vi "Process.vi"(8 "error in":errorcluster, 11 "Inst.Krohn-Hite-7008":refnum<class "Inst.Krohn-Hite-7008.lvclass">) -> (0 "error out":errorcluster, 3 "Inst.Krohn-Hite-7008 out":refnum<class "Inst.Krohn-Hite-7008.lvclass">)   [LabVIEW 2019, in "Inst.Krohn-Hite-7008.lvclass"]
doc: "---------------------------------------------------------------\nJKI State Machine Objects™\nhttp://jki.net/state-machine-objects/\nCopyright (C) 2005-2015, JKI <info@jki.net>\nALL RIGHTS RESERVED"
uses:
  Inst.Krohn-Hite-7008.lvclass
  C:/Program Files (x86)/National Instruments/LabVIEW 2019/vi.lib/JKI/JKI SMO/SMO/SMO.lvclass
  C:/Program Files (x86)/National Instruments/LabVIEW 2019/user.lib/LevyLab/Instrument Framework/Instrument/Instrument.lvclass
  Typedefs/Inst.Krohn-Hite-7008.Commands--Enum.ctl
  Typedefs/PrivateEvents--Inst.Krohn-Hite-7008.MessageToProcess.ctl
  <userlib>/LevyLab/RemoteControl/Typedefs/Message--Cluster.ctl
  <vilib>/JKI/JKI SMO/SMO/SMO.lvclass/SMO.ctl
  Inst.Krohn-Hite-7008.lvclass/Inst.Krohn-Hite-7008.ctl
  Typedefs/Inst.Krohn-Hite-7008.ProtectedCommands--Enum.ctl
  ef847fcc-ae38-4c9a-a9d7-f0d56e5c7fa0.vi
  c2686cc3-20e9-4710-a87a-2e2b9cb24138.vi
  <vilib>/JKI/JKI SMO/SMO/Private/ReftoDVR--SMO.vi
  <vilib>/Utility/Data Type/Get Type Information.vi
  <vilib>/Utility/Data Type/Get Numeric Information.vi
  <userlib>/_OpenG.lib/lvdata/lvdata.llb/Unwrap VVariant__ogtk.vi
  <userlib>/LevyLab/Instrument Framework/Instrument Types/Amplifier/Instrument.Amplifier.lvclass
  <vilib>/JKI/JKI SMO/SMO/SMO.lvclass
  <userlib>/LevyLab/Instrument Framework/Instrument/Instrument.lvclass
  <userlib>/LevyLab/RemoteControl/RemoteControl.lvclass
  KH7008/KH7008.lvlib
  <userlib>/LevyLab/Configuration/Debug.lvlib
panel:
  out "Status":string
  out "State History":string
  # "Instrument.Krohn-Hite-7008"
  # "Instrument.Krohn-Hite-7008"
  # "For instructions on how to use the JKI State Machine Objects, examples and video tutorials, visit:\nhttp://jki.net/state-machine-objects/\n\nJKI State Machine Objects™\nhttp://jki.net/state-machine-objects/\nCopyright (C) 2005-2015, JKI <info@jki.net>\nALL RIGHTS RESERVED"
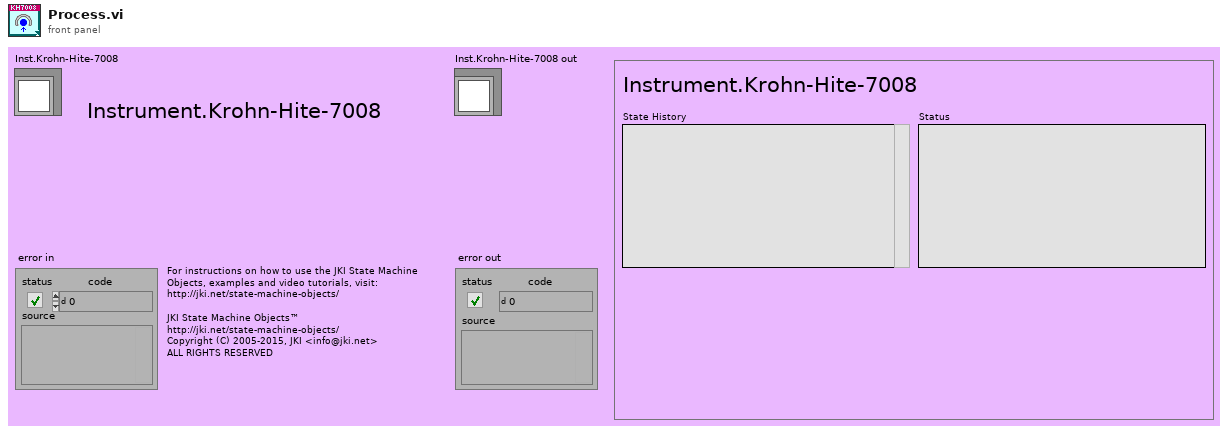
[diagram p1: front panel]
types:
  T1 = typedef "Inst.Krohn-Hite-7008.lvclass/Inst.Krohn-Hite-7008.Commands--Enum.ctl" = enum16{"getChannel", "getAllChannels", "setChannel", "setAllChannels"}
  T2 = enum32{"invalid app kind", "Development System", "Run Time System", "Student Edition", "Embedded LabVIEW", "Evaluation", "Custom"}
  T3 = enum32{"Invalid", "Standard", "Closed", "Hidden", "Minimized", "Maximized"}
  T4 = typedef "Inst.Krohn-Hite-7008.lvclass/Inst.Krohn-Hite-7008.ProtectedCommands--Enum.ctl" = enum16{"Update allChannelProperties", "Update device", "Set SR"}
  T5 = typedef "Inst.Krohn-Hite-7008.lvclass/PrivateEvents--Inst.Krohn-Hite-7008.MessageToProcess.ctl" = cluster{"Message":T6}
  T6 = typedef "RemoteControl.lvclass/Message--Cluster.ctl" = cluster{"Command":string, "Data":variant, "ID":string}
  T7 = cluster{"Core":cluster{"Current VI Reference":refnum<vi>, "Close Panel on Exit?":bool, "Last Error":cluster{"error":errorcluster, "previous state":string, "remaining states":string}, "Shutdown?":bool}, "SelfRef":refnum<class "Inst.Krohn-Hite-7008.lvclass">, "Running Step":i32, "sequence":string[], "MessageToProcess":T5, "UI Behavior":string, "wait":u32}
  T8 = cluster{"Current VI Reference":refnum<vi>, "Close Panel on Exit?":bool, "Last Error":cluster{"error":errorcluster, "previous state":string, "remaining states":string}, "Shutdown?":bool}
  T9 = typedef "Debug.lvlib/Attribute.Debug.lvclass/DebugBehavior.ctl" = enum16{"Normal", "Debug"}
  T10 = typedef "SMO.lvclass/Protected Events.ctl" = cluster{"StopProcesses":refnum<user-event>, "AbortProcesses":refnum<user-event>, "Config Changed":refnum<user-event>, "Dependency":refnum<user-event>}
  T11 = typedef "KH7008.lvlib/allChannelProperties--Array.ctl" = T12[]
  T12 = typedef "KH7008.lvlib/channelProperties--Cluster.ctl" = cluster{"channel":T13, "gain":T14, "input":T15, "shunt":T16, "couple":T17, "filter":T18}
  T13 = typedef "KH7008.lvlib/channel--numeric.ctl" = u16
  T14 = typedef "KH7008.lvlib/gain--enum.ctl" = enum16{"1", "10", "100", "1000"}
  T15 = typedef "KH7008.lvlib/input--enum.ctl" = enum16{"OFF", "SE+", "SE-", "DIFF"}
  T16 = typedef "KH7008.lvlib/shunt--enum.ctl" = enum16{"Open", "50", "500", "5k", "50k", "10M"}
  T17 = typedef "KH7008.lvlib/couple--enum.ctl" = enum16{"AC", "DC"}
  T18 = typedef "KH7008.lvlib/filter--enum.ctl" = enum16{"OFF", "ON"}
  T19 = typedef "Inst.Krohn-Hite-7008.lvclass/Inst.Krohn-Hite-7008.getAll--Cluster.ctl" = cluster{"device_id":string, "model":string, "allChannelProperties_json":string, "allChannelProperties":T11}
  T20 = typedef "Inst.Krohn-Hite-7008.lvclass/getAllChannelsDatabase--Cluster.ctl" = cluster{"device_id":string, "channel":u32, "gain":string, "input":string, "shunt":string, "couple":string, "filter":string}
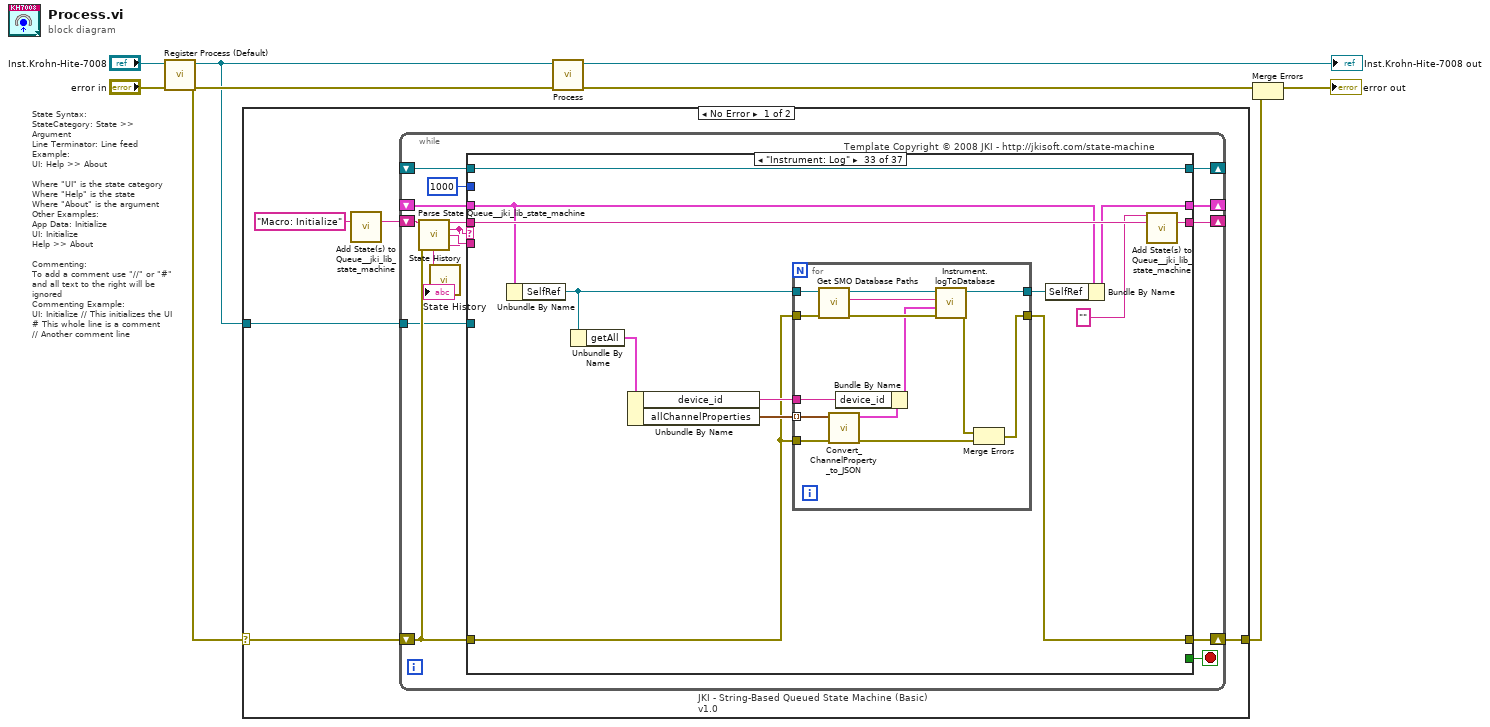
[diagram p0: block diagram]
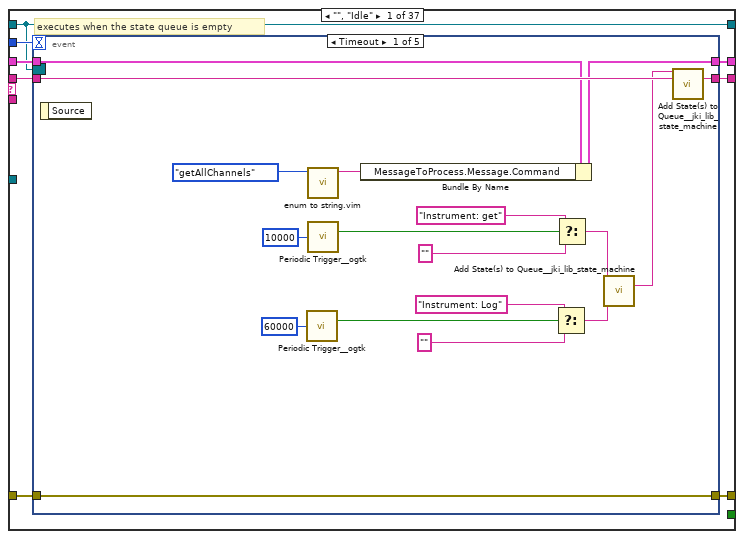
[diagram p2: hidden frame]
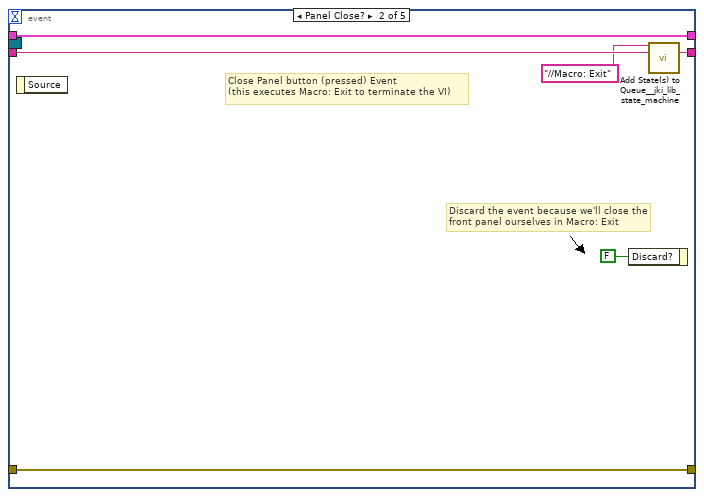
[diagram p3: hidden frame]
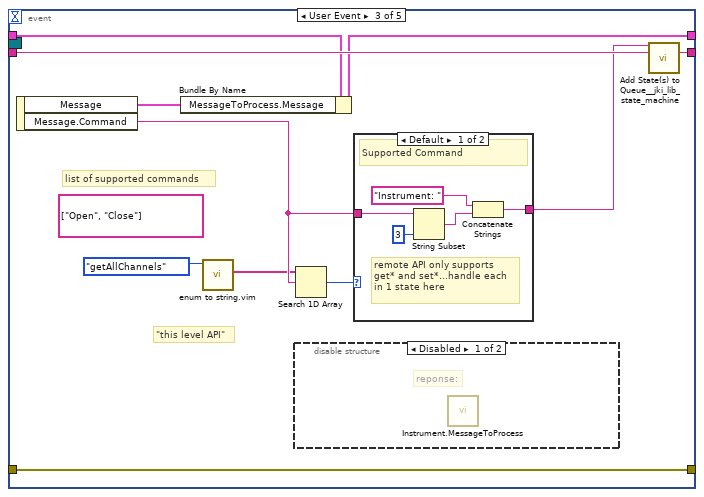
[diagram p4: hidden frame]
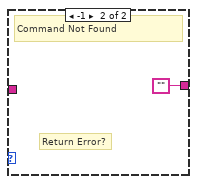
[diagram p6: hidden frame]
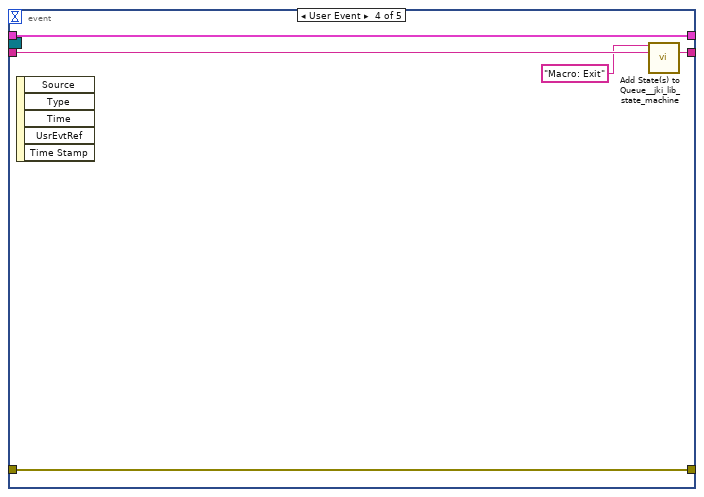
[diagram p7: hidden frame]
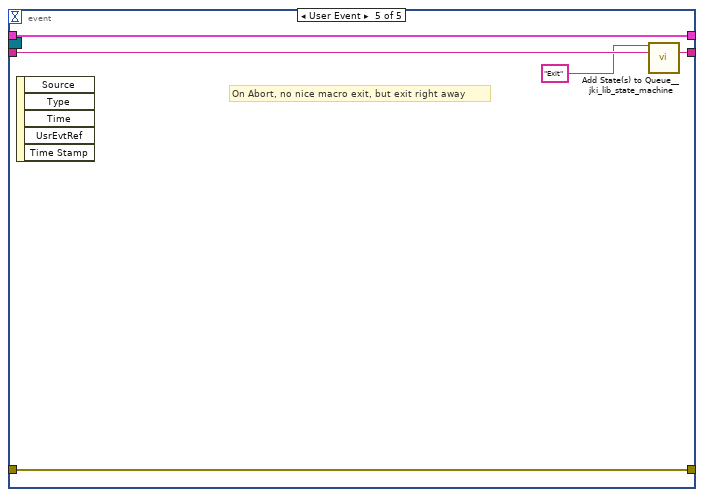
[diagram p8: hidden frame]
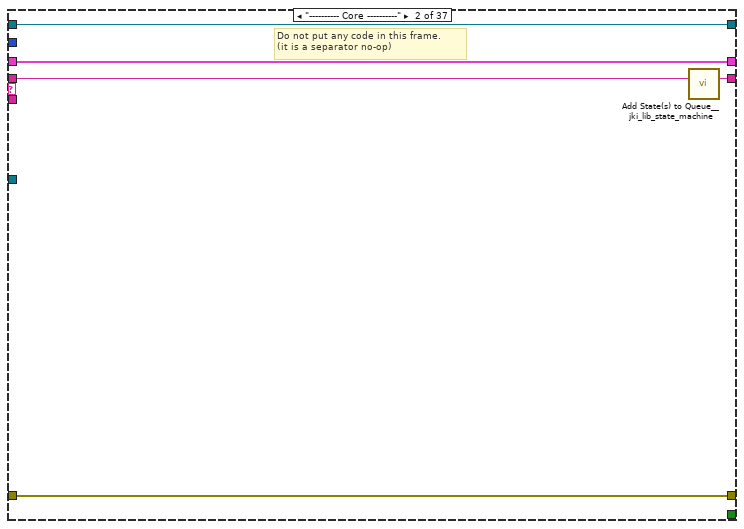
[diagram p9: hidden frame]
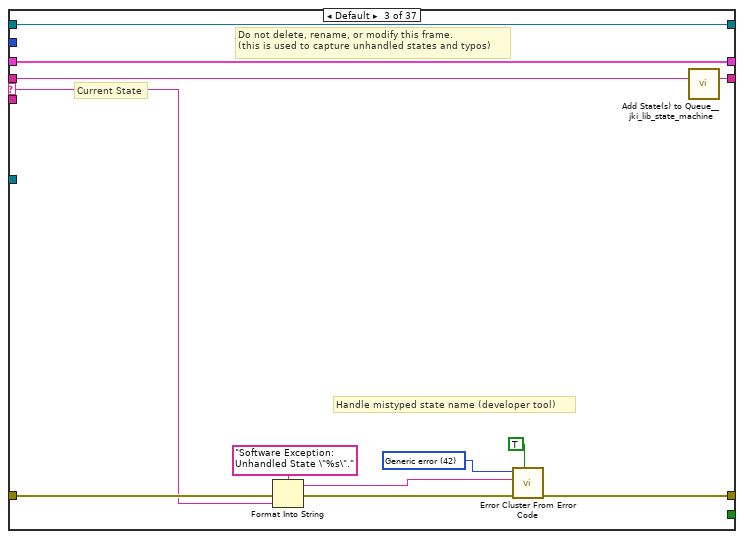
[diagram p10: hidden frame]
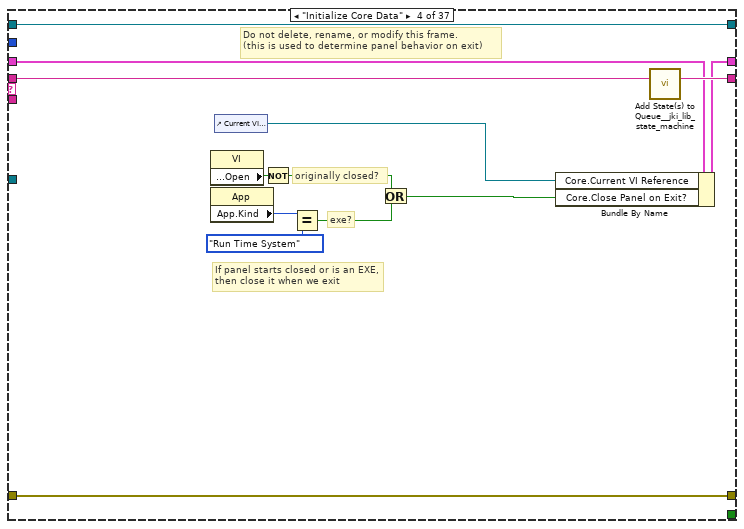
[diagram p11: hidden frame]
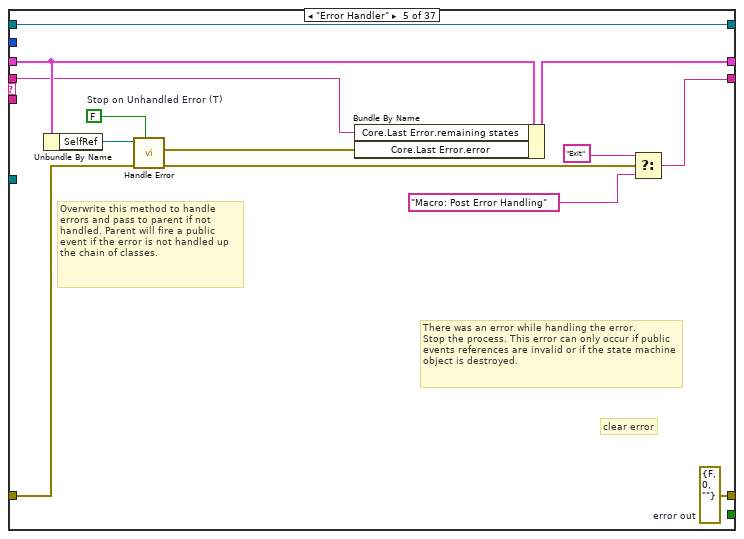
[diagram p12: hidden frame]
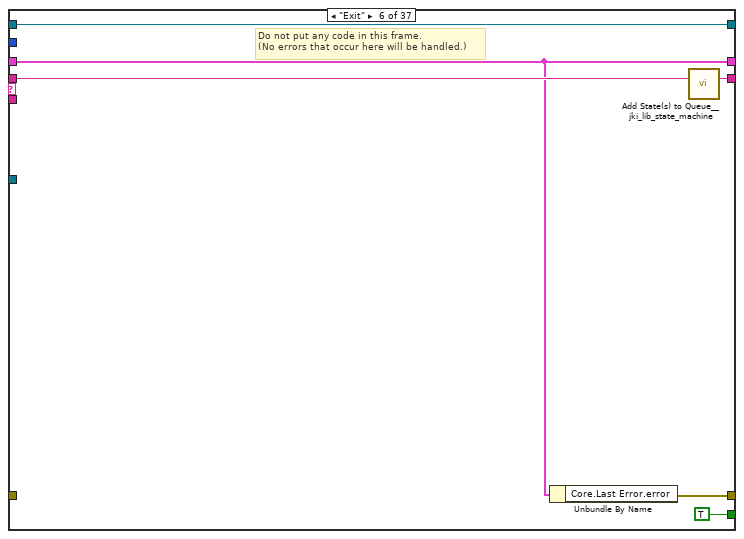
[diagram p13: hidden frame]
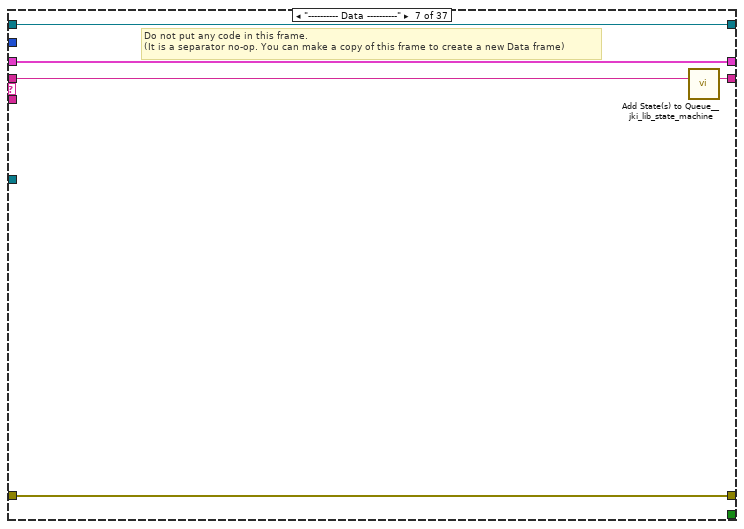
[diagram p14: hidden frame]
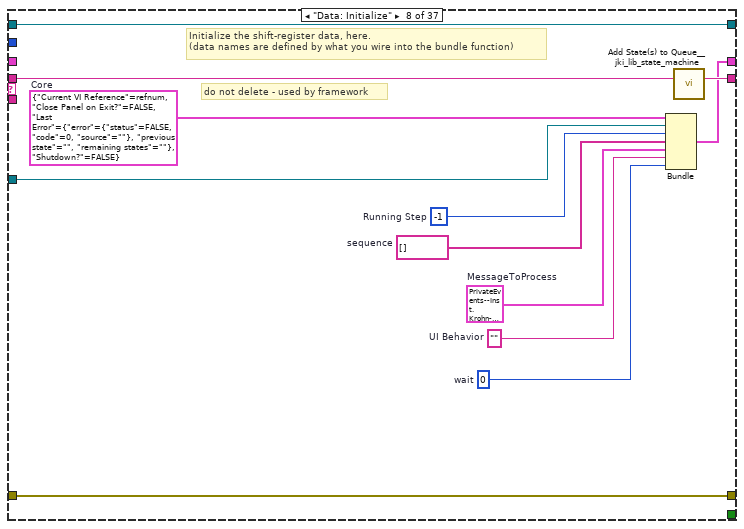
[diagram p15: hidden frame]
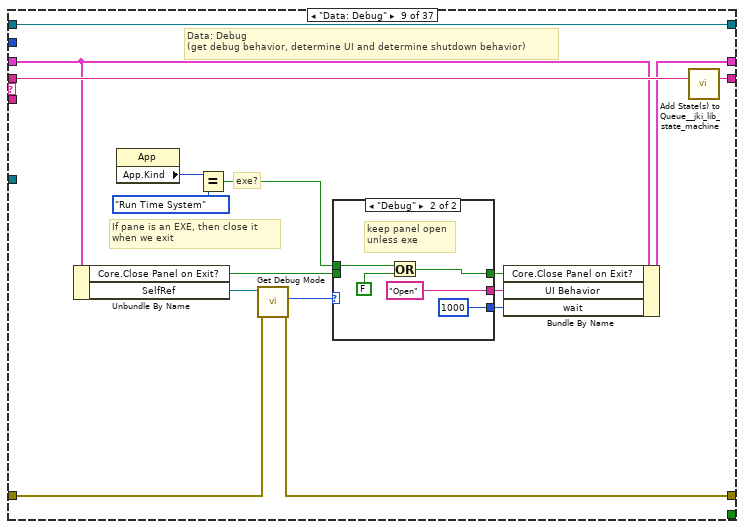
[diagram p16: hidden frame]
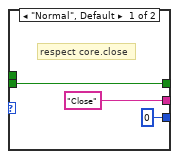
[diagram p17: hidden frame]
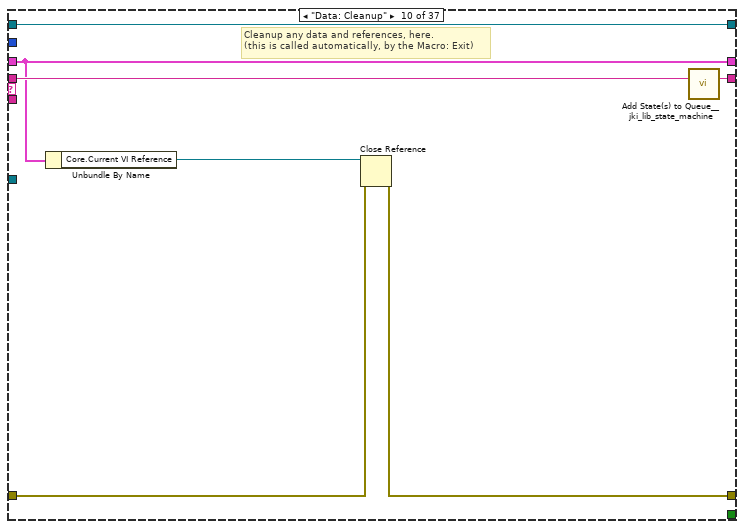
[diagram p18: hidden frame]
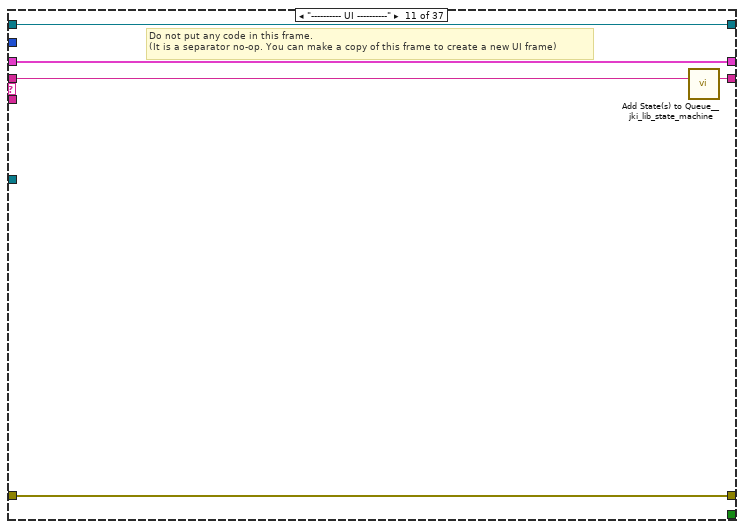
[diagram p19: hidden frame]
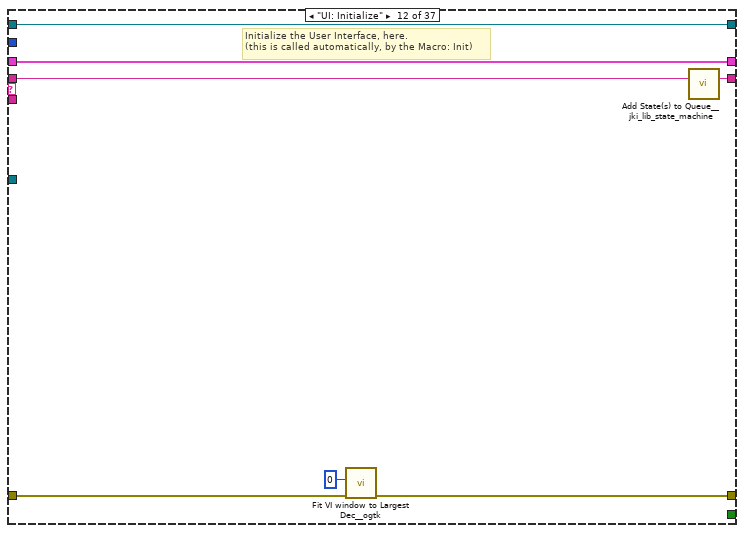
[diagram p20: hidden frame]
diagram:
  # "State Syntax:\nStateCategory: State >> Argument\nLine Terminator: Line feed\nExample:\nUI: Help >> About\n\nWhere \"UI\" is the state category\nWhere \"Help\" is the state\nWhere \"About\" is the argument\nOther Examples:\nApp Data: Initialize\nUI: Initialize\nHelp >> About\n\nCommenting:\nTo add a comment use \"//\" or \"#\" and all text to the right will be ignored\nCommenting Example:\nUI: Initialize // This initializes the UI\n# This whole line is a comment\n// Another comment line"
  n1 = call <vilib>:"Register Process (Default).vi"("error in (no error)"="error in", "SMO"="Inst.Krohn-Hite-7008") -> ("error out"=w5:errorcluster, "SelfRef"=w4:refnum<class "Inst.Krohn-Hite-7008.lvclass">)  [unwired: 8 in]
  n2 = case shown="No Error" w5 {
    selector: w5 -> [w10 w522]
    tunnel: w4 -> [w11 _]
    tunnel: [w9 w522] -> w1
    frame No Error {
      n3 = call <vilib>:"Add State(s) to Queue__jki_lib_state_machine.vi"("State(s) in (\"\")"="Macro: Initialize") -> ("States Out"=w13:string)  [unwired: 14 in]
      n4 = while "JKI - String-Based Queued State Machine (Basic) v1.0" {
        shift-right: [w22] -> _
        shift-left: _ -> [w21]
        shift-right: [w25] -> w9
        shift-left: w10 -> [w19]
        shift-right: [w24] -> _
        shift-left: w13 -> [w26]
        tunnel: w11 -> [w18]
        shift-right: [w17] -> _
        shift-left: _ -> [w16]
        stop <- w23 stop-if-true
        # "Template Copyright © 2008 JKI - http://jkisoft.com/state-machine"
        n5 = call <vilib>:"Parse State Queue__jki_lib_state_machine.vi"("State Queue"=w26, "Error In (no error)"=w19) -> ("Remaining States"=w28:string, "Current State"=w15:string, "Arguments"=w27:string)  [unwired: 11 in]
        n6 = call <userlib>:"State History.vi"("Current State"=w15) -> ("History"=→"State History":string)  [unwired: 10 in]
        n7 = case shown="\"Instrument: Log\"" w15 {
          selector: w15 -> [_ _ w94 _ _ _ _ _ _ _ _ _ _ _ _ _ _ _ _ _ _ _ _ _ _ _ _ _ _ _ _ _ _ _ _ _ _]
          tunnel: w28 -> [w36 w92 w98 w117 w122 w136 w141 w153 w169 w184 w189 w196 w203 w219 w251 w260 w268 w274 _ w317 w332 w337 w348 w355 w360 w373 w379 w386 w395 w409 w428 w455 w468 w491 w496 w502 w521]
          tunnel: w27 -> [_ _ _ _ _ _ _ _ _ _ _ _ w197 w213 _ _ _ _ _ _ _ _ _ _ _ _ _ _ _ _ _ _ _ _ _ w497 w505]
          tunnel: w21 -> [w34 w89 w96 w108 w126 w132 w138 _ w157 w179 w186 w194 w201 w215 w248 w257 w264 w271 w277 w307 w322 w334 w345 w352 w357 w366 w377 w381 w391 w405 w424 w451 w464 w487 w492 w498 w511]
          tunnel: [w33 w90 w100 w114 w127 w131 w139 w145 w156 w180 w187 w191 w198 w216 w249 w252 w266 w272 w285 w315 w318 w335 w339 w350 w358 w369 w375 w383 w388 w400 w420 w447 w459 w484 w493 w499 w513] -> w25
          tunnel: w19 -> [w32 w90 w99 w114 w128 _ w139 w145 w155 w181 w187 w190 w199 w217 w249 w252 w266 w272 w285 w315 w318 w335 w340 w349 w358 w363 w375 w383 w389 w399 w419 w448 w456 w483 w493 w499 w507]
          tunnel: [w35 w91 w97 w116 w118 w135 w140 w152 w168 w183 w188 w195 w202 w218 w250 w259 w267 w273 w286 w316 w331 w336 w347 w354 w359 w372 w378 w385 w394 w408 w427 w454 w467 w490 w495 w501 w520] -> w24
          tunnel: [_ _ _ _ _ TRUE _ _ _ _ _ _ _ _ _ _ _ _ _ _ _ _ _ _ _ _ _ _ _ _ _ _ _ _ _ _ _] -> w23
          tunnel: [w31 w89 w96 w115 w125 w132 w138 w151 w158 w179 w186 w194 w201 w215 w248 w257 w264 w271 w278 w308 w322 w334 w345 w352 w357 w366 w377 w382 w392 w406 w425 w452 w465 w488 w492 w498 w510] -> w22
          tunnel: 1000 ("Timeout") -> [w30 _ _ _ _ _ _ _ _ _ _ _ _ _ _ _ _ _ _ _ _ _ _ _ _ _ _ _ _ _ _ _ _ _ _ _ _]
          tunnel: w18 -> [_ _ _ _ _ _ _ w146 _ _ _ _ _ _ _ _ _ _ _ _ _ _ _ _ _ _ _ _ _ _ _ _ _ _ _ _ _]
          tunnel: [w29 w88 w93 w105 w130 w133 w137 w150 w167 w178 w185 w193 w200 w212 w247 w258 w265 w270 w284 w314 w327 w333 w346 w353 w356 w371 w376 w384 w393 w407 w426 w453 w466 w489 w494 w500 w519] -> w17
          tunnel: w16 -> [w29 w88 w93 w105 w130 w133 w137 w150 w167 w178 w185 w193 w200 w212 w247 w258 w265 w270 w284 w314 w327 w333 w346 w353 w356 _ w376 w384 w393 w407 w426 w453 w466 w489 w494 w500 w519]
          frame "", "Idle" {
            # "executes when the state queue is empty"
            n8 = event shown="[0] Timeout" {
              selector: w29 -> [_ _ _ _ _]
              dyn-events: _ -> [_ _ _ _ _]
              timeout: w30 -> [_ _ _ _ _]
              tunnel: w36 -> [w54 w60 w71 w82 w87]
              tunnel: [w53 w59 w70 w81 w86] -> w35
              tunnel: w34 -> [w48 w57 w64 w79 w84]
              tunnel: [w52 w58 w69 w80 w85] -> w33
              tunnel: w32 -> [w52 w58 w69 w80 w85]
              tunnel: [w49 w57 w65 w79 w84] -> w31
              event Timeout {
                n9 = event-data() -> ()  [unwired: 1 in, 1 out]
                n10 = call <userlib>:"Periodic Trigger__ogtk.vi"("time (ms)"=u32 60000) -> ("Triggered"=w40:bool)  [unwired: 12 in, 2 out]
                n11 = call "enum to string.vim"("enum in"=Inst.Krohn-Hite-7008.Commands--Enum."getAllChannels" ("Commands")) -> ("string out"=w51:string)  [unwired: 9 in, 1 out]
                n12 = call <userlib>:"Periodic Trigger__ogtk.vi"("time (ms)"=u32 10000) -> ("Triggered"=w47:bool)  [unwired: 12 in, 2 out]
                n13 = Bundle By Name(cluster=w48, "MessageToProcess.Message.Command"=w51) -> (w49:T7)
                n14 = Select(t="Instrument: Log", s=w40, f="") -> (s? t:f=w39:string)
                n15 = Select(t="Instrument: get", s=w47, f="") -> (s? t:f=w38:string)
                n16 = call <vilib>:"Add State(s) to Queue__jki_lib_state_machine.vi"("State(s) in Front (\"\")"=w38, "State(s) at Back (\"\")"=w39) -> ("States Out"=w37:string)  [unwired: 13 in]
                n17 = call <vilib>:"Add State(s) to Queue__jki_lib_state_machine.vi"("State(s) in Front (\"\")"=w37, "State(s) in (\"\")"=w54) -> ("States Out"=w53:string)  [unwired: 13 in]
              }
              event Panel Close? {
                # "Discard the event because we'll close the front panel ourselves in Macro: Exit"
                # "Close Panel button (pressed) Event\n(this executes Macro: Exit to terminate the VI)"
                n18 = event-data() -> ()  [unwired: 1 in, 1 out]
                n19 = event-data("Discard?"=FALSE) -> ()  [unwired: 1 in, 1 out]
                n20 = call <vilib>:"Add State(s) to Queue__jki_lib_state_machine.vi"("State(s) in Front (\"\")"="//Macro: Exit", "State(s) in (\"\")"=w60) -> ("States Out"=w59:string)  [unwired: 13 in]
              }
              event User Event {
                (unwired) string[] ["Open", "Close"]
                # "\"this level API\""
                # "list of supported commands"
                n21 = event-data() -> ("Message"=w63:T6, "Message.Command"=w66:string)  [unwired: 1 in]
                n22 = Bundle By Name(cluster=w64, "MessageToProcess.Message"=w63) -> (w65:T7)
                n23 = call "enum to string.vim"("enum in"=Inst.Krohn-Hite-7008.Commands--Enum."getAllChannels" ("Commands")) -> ("strings out"=w61:string[])  [unwired: 9 in, 1 out]
                n24 = disable-structure shown="Disabled" {
                  frame Disabled {
                    # "reponse:"
                    n25 = call <userlib>:"Instrument.MessageToProcess.vi"() -> ()  [unwired: 10 in, 2 out]
                  }
                  frame Enabled {
                  }
                }
                n26 = Search 1D Array(1D array=w61, element=w66) -> (index of element=w68:i32)  [unwired: 1 in]
                n27 = case shown="Default" w68 {
                  tunnel: [w76 "" ("Empty String Constant")] -> w67
                  tunnel: w66 -> [w72 _]
                  frame Default {
                    # "remote API only supports\nget* and set*...handle each \nin 1 state here"
                    # "Supported Command"
                    n28 = String Subset(string=w72, length (rest)=3 ("length (rest)")) -> (substring=w73:string)  [unwired: 1 in]
                    n29 = Concatenate Strings("Instrument: ", w73) -> (w76:string)
                  }
                  frame -1 {
                    # "Return Error?"
                    # "Command Not Found"
                  }
                }
                n30 = call <vilib>:"Add State(s) to Queue__jki_lib_state_machine.vi"("State(s) in Front (\"\")"=w67, "State(s) in (\"\")"=w71) -> ("States Out"=w70:string)  [unwired: 13 in]
              }
              event User Event {
                n31 = event-data() -> ()  [unwired: 1 in, 5 out]
                n32 = call <vilib>:"Add State(s) to Queue__jki_lib_state_machine.vi"("State(s) in Front (\"\")"="Macro: Exit", "State(s) in (\"\")"=w82) -> ("States Out"=w81:string)  [unwired: 13 in]
              }
              event User Event {
                # "On Abort, no nice macro exit, but exit right away"
                n33 = event-data() -> ()  [unwired: 1 in, 5 out]
                n34 = call <vilib>:"Add State(s) to Queue__jki_lib_state_machine.vi"("State(s) in Front (\"\")"="Exit", "State(s) in (\"\")"=w87) -> ("States Out"=w86:string)  [unwired: 13 in]
              }
            }
          }
          frame "---------- Core ----------" {
            # "Do not put any code in this frame.\n(it is a separator no-op)"
            n35 = call <vilib>:"Add State(s) to Queue__jki_lib_state_machine.vi"("State(s) in (\"\")"=w92) -> ("States Out"=w91:string)  [unwired: 14 in]
          }
          frame Default {
            w103 = 42 items=["No error", "Argument error", "Memory is full", "Out of zone", "End of file", "File already open", "Generic file I/O error", "File not found", "File permission error", "Disk is full", "Duplicate path", "Too many files open", "System feature not enabled", "Resource file not found", "Cannot add resource", "Resource not found", "Image not found", "Image memory error", "Pen does not exist", "Config type invalid", "Config token not found", "Config parse error", "Config memory error", "Bad external code format", "Bad external code offset", "External code not present", "Null window", "Destroy window error", "Null menu", "Print aborted", "Bad print record", "Print driver error", "Windows error during printing", "Memory error during printing", "Print dialog error", "Generic print error", "Invalid device refnum", "Device not found", "Device parameter error", "Device unit error", "Cannot open device", "Device call aborted", "Generic error", "Cancelled by user", "Object ID too low", "Object ID too high", "Object not in heap", "Unknown heap", "Unknown object (invalid DefProc)", "Unknown object (DefProc not in table)", "Message out of range", "Invalid (null) method", "Unknown message", "Manager call not supported", "Bad address", "Network operation in progress", "Network operation timed out", "Connection is busy", "Network attribute not supported", "Network error", "Address in use", "System out of memory", "Connection aborted", "Connection refused", "Not connected", "Already connected", "Connection closed", "Initialization error (interapplication manager)", "Bad occurrence", "Wait on unbound occurrence handler", "Occurrence queue overflow", "Datalog type conflict", "Unused", "Unrecognized type (interapplication manager)", "Memory corrupt", "Failed to make temporary DLL", "Old CIN version", "Drag socket not found", "Failed to load drop-object", "Failed to register OLE object", "Failed to release OLE object", "Format specifier type mismatch", "Unknown format specifier", "Too few format specifiers", "Too many format specifiers", "Scan failed", "Newer CIN version", "Error converting to variant", "Runtime menu error", "Password tampered", "Variant attribute not found", "Incompatible variant data type", "Event data is not available", "Event Store is not present", "Occurrence is not found", "Event Queue is not created", "Event info is not available", "Refnum passed is NULL", "Error retrieving Class GUID", "Error retrieving CoClass GUID", "Error retrieving TypeLib GUID.", "Bad built application magic bytes.", "Specific driver is different from the specific driver associated with the Logical Name.", "There is no session opened to the class driver.", "Max Error", "MAX - Error with config objects", "MAX - Error loading configuration", "MAX - Group not supported"]
            # "Current State"
            # "Do not delete, rename, or modify this frame.\n(this is used to capture unhandled states and typos)"
            # "Handle mistyped state name (developer tool)"
            n36 = Format Into String(format string="Software Exception: Unhandled State \"%s\"." ("message"), error in=w99, w94) -> (resulting string=w102:string, error out=w101:errorcluster)  [unwired: 1 in]
            n37 = call <vilib>:"Error Cluster From Error Code.vi"("show call chain? (False)"=TRUE, "error in (no error)"=w101, "error message (\"\")"=w102, "error code (0)"=w103) -> ("error out"=w100:errorcluster)  [unwired: 5 in]
            n38 = call <vilib>:"Add State(s) to Queue__jki_lib_state_machine.vi"("State(s) in (\"\")"=w98) -> ("States Out"=w97:string)  [unwired: 14 in]
          }
          frame "Initialize Core Data" {
            # "Do not delete, rename, or modify this frame.\n(this is used to determine panel behavior on exit)"
            # "originally closed?"
            # "exe?"
            # "If panel starts closed or is an EXE, then close it when we exit"
            n39 = property class="VI"() -> ("Front Panel.Open"=w113:bool)  [unwired: 2 in, 2 out]
            n40 = property class="App"() -> ("App.Kind"=w112:T2)  [unwired: 2 in, 2 out]
            n41 = control-ref of="Current VI Reference"() -> (w106:refnum<vi>)
            n42 = Not(x=w113) -> (.not. x?=w110:bool)
            n43 = Equal?(x=w112, y=T2."Run Time System" ("Application:Kind")) -> (x = y?=w109:bool)
            n44 = Or(x=w110, y=w109) -> (x .or. y?=w107:bool)
            n45 = Bundle By Name(cluster=w108, "Core.Current VI Reference"=w106, "Core.Close Panel on Exit?"=w107) -> (w115:T7)
            n46 = call <vilib>:"Add State(s) to Queue__jki_lib_state_machine.vi"("State(s) in (\"\")"=w117) -> ("States Out"=w116:string)  [unwired: 14 in]
          }
          frame "Error Handler" {
            w123 = FALSE  # Stop on Unhandled Error (T)
            w127 = errorcluster {"status"=FALSE, "code"=0, "source"=""}  # error out
            # "clear error"
            # "There was an error while handling the error.\nStop the process. This error can only occur if public events references are invalid or if the state machine object is destroyed."
            # "Overwrite this method to handle errors and pass to parent if not handled. Parent will fire a public event if the error is not handled up the chain of classes."
            n47 = Unbundle By Name(w126) -> ("SelfRef"=w129:refnum<class "Inst.Krohn-Hite-7008.lvclass">)
            n48 = call-dynamic "Handle Error.vi"("Stop on Unhandled Error (T)"=w123, "error in"=w128, "SMO"=w129) -> ("handling error"=w119:errorcluster, "Unhandled error"=w124:errorcluster)  [unwired: 6 in, 1 out]
            n49 = Bundle By Name(cluster=w126, "Core.Last Error.remaining states"=w122, "Core.Last Error.error"=w124) -> (w125:T7)
            n50 = Select(t="Exit", s=w119, f="Macro: Post Error Handling") -> (s? t:f=w118:string)
          }
          frame "Exit" {
            # "Do not put any code in this frame.\n(No errors that occur here will be handled.)"
            n51 = Unbundle By Name(w132) -> ("Core.Last Error.error"=w131:errorcluster)
            n52 = call <vilib>:"Add State(s) to Queue__jki_lib_state_machine.vi"("State(s) in (\"\")"=w136) -> ("States Out"=w135:string)  [unwired: 14 in]
          }
          frame "---------- Data ----------" {
            # "Do not put any code in this frame.\n(It is a separator no-op. You can make a copy of this frame to create a new Data frame)"
            n53 = call <vilib>:"Add State(s) to Queue__jki_lib_state_machine.vi"("State(s) in (\"\")"=w141) -> ("States Out"=w140:string)  [unwired: 14 in]
          }
          frame "Data: Initialize" {
            w142 = u32 0  # wait
            w143 = ""  # UI Behavior
            w144 = T5 {"Message"={"Command"="", "Data"=variant(string ""), "ID"=""}}  # MessageToProcess
            w147 = string[] []  # sequence
            w148 = -1  # Running Step
            w149 = T8 {"Current VI Reference"=refnum, "Close Panel on Exit?"=FALSE, "Last Error"={"error"={"status"=FALSE, "code"=0, "source"=""}, "previous state"="", "remaining states"=""}, "Shutdown?"=FALSE}  # Core
            # "do not delete - used by framework"
            # "Initialize the shift-register data, here.\n(data names are defined by what you wire into the bundle function)"
            n54 = Bundle("Core"=w149, "SelfRef"=w146, "Running Step"=w148, "sequence"=w147, "MessageToProcess"=w144, "UI Behavior"=w143, "wait"=w142) -> (w151:T7)  [unwired: 1 in]
            n55 = call <vilib>:"Add State(s) to Queue__jki_lib_state_machine.vi"("State(s) in (\"\")"=w153) -> ("States Out"=w152:string)  [unwired: 14 in]
          }
          frame "Data: Debug" {
            # "exe?"
            # "If pane is an EXE, then close it when we exit"
            # "Data: Debug\n(get debug behavior, determine UI and determine shutdown behavior)"
            n56 = Unbundle By Name(w157) -> ("Core.Close Panel on Exit?"=w160:bool, "SelfRef"=w166:refnum<class "Inst.Krohn-Hite-7008.lvclass">)
            n57 = property class="App"() -> ("App.Kind"=w163:T2)  [unwired: 2 in, 2 out]
            n58 = Equal?(x=w163, y=T2."Run Time System" ("Application:Kind")) -> (x = y?=w159:bool)
            n59 = call <userlib>:"Get Debug Mode.vi"("error in (no error)"=w155, "SMO"=w166) -> ("error out"=w156:errorcluster, "Behavior"=w165:T9)  [unwired: 7 in, 1 out]
            n60 = case shown="\"Debug\"" w165 {
              tunnel: ["Close" "Open"] -> w164
              tunnel: [u32 0 ("wait") u32 1000 ("wait")] -> w154
              tunnel: [w170 w173] -> w161
              tunnel: w160 -> [w170 _]
              tunnel: w159 -> [_ w175]
              frame "Normal", Default {
                # "respect core.close"
              }
              frame "Debug" {
                # "keep panel open\nunless exe"
                n61 = Or(x=w175, y=FALSE) -> (x .or. y?=w173:bool)
              }
            }
            n62 = Bundle By Name(cluster=w157, "Core.Close Panel on Exit?"=w161, "UI Behavior"=w164, "wait"=w154) -> (w158:T7)
            n63 = call <vilib>:"Add State(s) to Queue__jki_lib_state_machine.vi"("State(s) in (\"\")"=w169) -> ("States Out"=w168:string)  [unwired: 14 in]
          }
          frame "Data: Cleanup" {
            # "Cleanup any data and references, here.\n(this is called automatically, by the Macro: Exit)"
            n64 = Unbundle By Name(w179) -> ("Core.Current VI Reference"=w182:refnum<vi>)
            n65 = Close Reference(reference=w182, error in (no error)=w181) -> (error out=w180:errorcluster)
            n66 = call <vilib>:"Add State(s) to Queue__jki_lib_state_machine.vi"("State(s) in (\"\")"=w184) -> ("States Out"=w183:string)  [unwired: 14 in]
          }
          frame "---------- UI ----------" {
            # "Do not put any code in this frame.\n(It is a separator no-op. You can make a copy of this frame to create a new UI frame)"
            n67 = call <vilib>:"Add State(s) to Queue__jki_lib_state_machine.vi"("State(s) in (\"\")"=w189) -> ("States Out"=w188:string)  [unwired: 14 in]
          }
          frame "UI: Initialize" {
            # "Initialize the User Interface, here.\n(this is called automatically, by the Macro: Init)"
            n68 = call <userlib>:"Fit VI window to Largest Dec__ogtk.vi"("error in (no error)"=w190, "border spacing (2 px)"=0) -> ("error out"=w191:errorcluster)  [unwired: 4 in, 1 out]
            n69 = call <vilib>:"Add State(s) to Queue__jki_lib_state_machine.vi"("State(s) in (\"\")"=w196) -> ("States Out"=w195:string)  [unwired: 14 in]
          }
          frame "UI: Cursor Set" {
            # "Argument"
            # "Initialize the User Interface, here.\n(this is called automatically, by the Macro: Init)"
            n70 = disable-structure shown="Default" {
              disable-tunnel: w199 -> [w204 w207]
              disable-tunnel: [w204 w206] -> w198
              disable-tunnel: w197 -> [_ w205]
              frame condition #0 {
              }
              frame condition #1 (active) {
                n71 = case shown="\"Idle\", Default" w205 {
                  tunnel: w207 -> [w209 w211]
                  tunnel: [w208 w210] -> w206
                  frame "Idle", Default {
                    n72 = call <vilib>:"Unset Busy.vi"("error in (no error)"=w209) -> ("error out"=w208:errorcluster)  [unwired: 10 in]
                  }
                  frame "Busy" {
                    n73 = call <vilib>:"Set Busy.vi"("error in (no error)"=w211) -> ("error out"=w210:errorcluster)  [unwired: 9 in, 1 out]
                  }
                }
              }
            }
            n74 = call <vilib>:"Add State(s) to Queue__jki_lib_state_machine.vi"("State(s) in (\"\")"=w203) -> ("States Out"=w202:string)  [unwired: 14 in]
          }
          frame "UI: Front Panel State" {
            # "Argument"
            # "Set Front Panel Open or Closed\n(Usage: \"UI: Front Panel State >> Open|Close\")"
            n75 = Unbundle By Name(w215) -> ("Core.Current VI Reference"=w214:refnum<vi>)
            n76 = disable-structure shown="Default" {
              disable-tunnel: w217 -> [w223 w246]
              disable-tunnel: [w222 w246] -> w216
              disable-tunnel: w214 -> [w221 _]
              disable-tunnel: w213 -> [w220 _]
              frame condition #0 (active) {
                n77 = case shown="\"Close\"" w220 {
                  tunnel: w223 -> [w227 w240]
                  tunnel: [w229 w241] -> w222
                  tunnel: w221 -> [w228 w238]
                  frame "Open", Default {
                    n78 = property class="VI"(reference=w228, error in=w227) -> (reference out=w225:refnum<vi>, error out=w226:errorcluster, "FP.State"=w224:T3)
                    n79 = case shown="\"Closed\"" w224 {
                      tunnel: [w232 w235] -> w229
                      tunnel: w226 -> [w231 w235]
                      tunnel: w225 -> [w230 _]
                      frame "Closed" {
                        n80 = invoke class="VI" method="FP.Open"(reference=w230, error in=w231, "Activate"=TRUE, "State"=T3."Standard") -> (error out=w232:errorcluster)  [unwired: 1 in, 4 out]
                      }
                      frame Default {
                      }
                    }
                  }
                  frame "Close" {
                    n81 = property class="VI"(reference=w238, error in=w240) -> (reference out=w237:refnum<vi>, error out=w239:errorcluster, "FP.State"=w236:T3)
                    n82 = case shown="Default" w236 {
                      tunnel: [w242 w245] -> w241
                      tunnel: w239 -> [w242 w244]
                      tunnel: w237 -> [_ w243]
                      frame "Invalid", "Closed" {
                      }
                      frame Default {
                        n83 = invoke class="VI" method="FP.Close"(reference=w243, error in=w244) -> (error out=w245:errorcluster)  [unwired: 1 in, 2 out]
                      }
                    }
                  }
                }
              }
              frame condition #1 {
              }
            }
            n84 = call <vilib>:"Add State(s) to Queue__jki_lib_state_machine.vi"("State(s) in (\"\")"=w219) -> ("States Out"=w218:string)  [unwired: 14 in]
          }
          frame "---------- Macro ----------" {
            # "Do not put any code in this frame.\n(It is a separator no-op. You can make a copy of this frame to create a new Macro frame)"
            n85 = call <vilib>:"Add State(s) to Queue__jki_lib_state_machine.vi"("State(s) in (\"\")"=w251) -> ("States Out"=w250:string)  [unwired: 14 in]
          }
          frame "Macro: Initialize" {
            # "Initialization Macro\n(This is called once, when the VI starts)"
            n86 = call <vilib>:"Add State(s) to Queue__jki_lib_state_machine.vi"("State(s) in Front (\"\")"="Data: Initialize\nInitialize Core Data\nEvents: Register", "State(s) in (\"\")"="Process: Sync", "State(s) at Back (\"\")"="UI: Initialize\nUI: Front Panel State >> Close\nMacro: Debug\nMacro: Initialize KH") -> ("States Out"=w255:string)  [unwired: 12 in]
            n87 = call <vilib>:"Add State(s) to Queue__jki_lib_state_machine.vi"("State(s) in Front (\"\")"=w255, "State(s) in (\"\")"=w260) -> ("States Out"=w259:string)  [unwired: 13 in]
          }
          frame "Macro: Debug" {
            n88 = Unbundle By Name(w264) -> ("UI Behavior"=w263:string)
            n89 = Format Into String(format string="Data: Debug\nUI: Front Panel State >> %s\n//Sequence: Wait", w263) -> (resulting string=w262:string)  [unwired: 2 in, 1 out]
            n90 = call <vilib>:"Add State(s) to Queue__jki_lib_state_machine.vi"("State(s) in Front (\"\")"=w262, "State(s) in (\"\")"=w268) -> ("States Out"=w267:string)  [unwired: 13 in]
          }
          frame "Macro: Initialize KH" {
            # "Do not put any code in this frame.\n(It is a separator no-op. You can make a copy of this frame to create a new Macro frame)"
            n91 = call <vilib>:"Add State(s) to Queue__jki_lib_state_machine.vi"("State(s) in Front (\"\")"="Instrument: Open Hardware\nInstrument: Get SR\nInstrument: get" ("State(s) in Front (\"\")"), "State(s) in (\"\")"=w274) -> ("States Out"=w273:string)  [unwired: 13 in]
          }
          frame "Macro: Post Error Handling" {
            # "Clear Last Error?"
            n92 = Unbundle By Name(w277) -> ("Core.Last Error.error"=w276:errorcluster, "Core.Last Error.remaining states"=w279:string, "Core.Shutdown?"=w280:bool)
            n93 = Unbundle By Name(w277) -> ("Core.Last Error.error"=w283:errorcluster)
            n94 = case shown="False" FALSE {
              tunnel: w283 -> [w300 _]
              tunnel: [w300 _] -> w282
              frame False {
              }
              frame True {
              }
            }
            n95 = case shown="False" w280 {
              tunnel: w279 -> [w289 w299]
              tunnel: [w288 w298] -> w275
              tunnel: w276 -> [w292 _]
              frame False {
                # "These are the remaining states (at the moment the error occured). States can be altered according to business logic."
                # "NOT SHUTTING DOWN"
                n96 = call <vilib>:"Clear Errors.vi"("error in (no error)"=w292, "specific error code to clear (0: all)"=-9873) -> ("error out"=w287:errorcluster, "specific error cleared?"=w290:bool)  [unwired: 4 in]
                n97 = case shown="True" w290 {
                  tunnel: w289 -> [w293 _]
                  tunnel: [w293 w297] -> w288
                  tunnel: w287 -> [_ _]
                  frame False {
                  }
                  frame True {
                    n98 = call "Device Error Dialog.vi"() -> ("retry?"=w295:bool)  [unwired: 11 in]
                    n99 = Select(t="Macro: Initialize KH", s=w295, f="Macro: Exit") -> (s? t:f=w297:string)
                  }
                }
              }
              frame True {
                # "Developer can decide to alter the states but should be aware that during the shutdown process, there are certain states that must be run for the SMO to properly shut itself (and this process) down. As such, one can add states to perform additional clean-ups, but should append the remaining state to be executed."
                # "SHUTTING DOWN"
                n100 = call <vilib>:"Add State(s) to Queue__jki_lib_state_machine.vi"("State(s) in (\"\")"=w299) -> ("States Out"=w298:string)  [unwired: 14 in]
              }
            }
            n101 = Bundle By Name(cluster=w277, "Core.Last Error.error"=w282) -> (w278:T7)
            n102 = call <vilib>:"Add State(s) to Queue__jki_lib_state_machine.vi"("State(s) in (\"\")"=w275) -> ("States Out"=w286:string)  [unwired: 14 in]
          }
          frame "Macro: Run Sequence" {
            # "0,1,2,3,4,"
            # "5"
            # "Do not put any code in this frame.\n(It is a separator no-op. You can make a copy of this frame to create a new Macro frame)"
            n103 = Unbundle By Name(w307) -> ("sequence"=w303:string[], "Running Step"=w301:i32)
            n104 = Array Size(array=w303) -> (size(s)=w313:i32)
            n105 = Index Array(array=w303, index=w301) -> (element=w302:string)
            n106 = Greater Or Equal?(x=w313, y=w301) -> (x >= y?=w305:bool)
            n107 = Select(t=-1 ("Running Step"), s=w305, f=w301) -> (s? t:f=w312:i32)
            n108 = Bundle By Name(cluster=w307, "Running Step"=w312) -> (w308:T7)
            n109 = Select(t="Sequence: Status >> ...", s=w305, f="Idle //Check Event Structure\nMacro: Run Sequence" ("State(s) at Back (\"\")")) -> (s? t:f=w304:string)
            n110 = call <vilib>:"Add State(s) to Queue__jki_lib_state_machine.vi"("State(s) in Front (\"\")"=w302, "State(s) at Back (\"\")"=w304) -> ("States Out"=w306:string)  [unwired: 13 in]
            n111 = call <vilib>:"Add State(s) to Queue__jki_lib_state_machine.vi"("State(s) in Front (\"\")"=w306, "State(s) in (\"\")"=w317) -> ("States Out"=w316:string)  [unwired: 13 in]
          }
          frame "Macro: Exit" {
            # "Exit Macro\n(This is called once, when the VI exits)"
            n112 = Unbundle By Name(w322) -> ("Core.Close Panel on Exit?"=w320:bool)
            n113 = Select(t="UI: Front Panel State >> Close", s=w320, f="" ("Empty String Constant")) -> (s? t:f=w329:string)
            n114 = call <vilib>:"Add State(s) to Queue__jki_lib_state_machine.vi"("State(s) in Front (\"\")"="Data: Cleanup\nEvents: Unregister\nProcess: SelfTerminate", "State(s) in (\"\")"="Process: Sync", "State(s) at Back (\"\")"="Exit") -> ("States Out"=w324:string)  [unwired: 12 in]
            n115 = call <vilib>:"Add State(s) to Queue__jki_lib_state_machine.vi"("State(s) in Front (\"\")"="Instrument: Close Hardware", "State(s) in (\"\")"=w329, "State(s) at Back (\"\")"=w324) -> ("States Out"=w328:string)  [unwired: 12 in]
            n116 = call <vilib>:"Add State(s) to Queue__jki_lib_state_machine.vi"("State(s) in Front (\"\")"=w328, "State(s) in (\"\")"=w332) -> ("States Out"=w331:string)  [unwired: 13 in]
          }
          frame "---------- Process ----------" {
            # "Template Separator\n(You can make a copy of, or modify, this frame)"
            n117 = call <vilib>:"Add State(s) to Queue__jki_lib_state_machine.vi"("State(s) in (\"\")"=w337) -> ("States Out"=w336:string)  [unwired: 14 in]
          }
          frame "Process: Sync" {
            n118 = Unbundle By Name(w345) -> ("SelfRef"=w341:refnum<class "Inst.Krohn-Hite-7008.lvclass">)
            n119 = call <vilib>:"WaitOnProcessSync.vi"("error in (no error)"=w340, "SMO"=w341) -> ("error out"=w339:errorcluster, "Don't run?"=w344:bool)  [unwired: 7 in, 1 out]
            n120 = Select(t="Data: Cleanup\nEvents: Unregister\nExit", s=w344, f="" ("Empty String Constant")) -> (s? t:f=w338:string)
            n121 = call <vilib>:"Add State(s) to Queue__jki_lib_state_machine.vi"("State(s) in Front (\"\")"=w338, "State(s) in (\"\")"=w348) -> ("States Out"=w347:string)  [unwired: 13 in]
          }
          frame "Process: SelfTerminate" {
            # "Process: SelfTerminate\n(You can make a copy of, or modify, this frame)"
            n122 = Unbundle By Name(w352) -> ("SelfRef"=w351:refnum<class "Inst.Krohn-Hite-7008.lvclass">)
            n123 = call <vilib>:"SelfTerminate.vi"("error in (no error)"=w349, "SMO in"=w351) -> ("error out"=w350:errorcluster)  [unwired: 8 in, 1 out]
            n124 = call <vilib>:"Add State(s) to Queue__jki_lib_state_machine.vi"("State(s) in (\"\")"=w355) -> ("States Out"=w354:string)  [unwired: 14 in]
          }
          frame "---------- Events ----------" {
            # "Template Separator\n(You can make a copy of, or modify, this frame)"
            n125 = call <vilib>:"Add State(s) to Queue__jki_lib_state_machine.vi"("State(s) in (\"\")"=w360) -> ("States Out"=w359:string)  [unwired: 14 in]
          }
          frame "Events: Register" {
            n126 = Unbundle By Name(w366) -> ("SelfRef"=w367:refnum<class "Inst.Krohn-Hite-7008.lvclass">)
            n127 = call <vilib>:"GetProtectedEvents.vi"("SMO"=w367) -> ("error out"=w365:errorcluster, "SMO Protected Events"=w370:T10, "SMO out"=w364:refnum<class "Inst.Krohn-Hite-7008.lvclass">)  [unwired: 8 in]
            n128 = call "Inst.Krohn-Hite-7008.GetPrivateEvents.vi"("Inst.Krohn-Hite-7008 in"=w364) -> ("error out"=w361:errorcluster, "Inst.Krohn-Hite-7008 Private Events"=w362:cluster{"MessageToProcess":refnum<user-event>})  [unwired: 8 in, 1 out]
            n129 = register-events(w370, w362) -> (reference out=w371:refnum<event-registration>, error out=w368:errorcluster)  [unwired: 2 in]
            n130 = Merge Errors(w368, w361, w365, w363) -> (w369:errorcluster)
            n131 = call <vilib>:"Add State(s) to Queue__jki_lib_state_machine.vi"("State(s) in (\"\")"=w373) -> ("States Out"=w372:string)  [unwired: 14 in]
          }
          frame "Events: Unregister" {
            n132 = Unregister For Events(event registration refnum=w376, error in=w375) -> (error out=w374:errorcluster)
            n133 = call <vilib>:"Clear Errors.vi"("error in (no error)"=w374) -> ()  [unwired: 5 in, 2 out]
            n134 = call <vilib>:"Add State(s) to Queue__jki_lib_state_machine.vi"("State(s) in (\"\")"=w379) -> ("States Out"=w378:string)  [unwired: 14 in]
          }
          frame "---------- Instrument ----------" {
            n135 = Unbundle By Name(w381) -> ("SelfRef"=w380:refnum<class "Inst.Krohn-Hite-7008.lvclass">)
            n136 = Bundle By Name(cluster=w381, "SelfRef"=w380) -> (w382:T7)
            n137 = call <vilib>:"Add State(s) to Queue__jki_lib_state_machine.vi"("State(s) in (\"\")"=w386) -> ("States Out"=w385:string)  [unwired: 14 in]
          }
          frame "Instrument: Open Hardware" {
            n138 = Unbundle By Name(w391) -> ("SelfRef"=w390:refnum<class "Inst.Krohn-Hite-7008.lvclass">)
            n139 = call-dynamic "Open Hardware.vi"("error in (no error)"=w389, "Inst.Krohn-Hite-7008 in"=w390) -> ("error out"=w388:errorcluster, "Inst.Krohn-Hite-7008 out"=w387:refnum<class "Inst.Krohn-Hite-7008.lvclass">)  [unwired: 8 in]
            n140 = Bundle By Name(cluster=w391, "SelfRef"=w387) -> (w392:T7)
            n141 = call <vilib>:"Add State(s) to Queue__jki_lib_state_machine.vi"("State(s) in (\"\")"=w395) -> ("States Out"=w394:string)  [unwired: 14 in]
          }
          frame "Instrument: Get SR" {
            n142 = Unbundle By Name(w405) -> ("SelfRef"=w403:refnum<class "Inst.Krohn-Hite-7008.lvclass">)
            n143 = Unbundle By Name(w403) -> ("VISA resource"=w404:refnum<visa-resource-name>)
            n144 = call "Get Installed SR Type.vi"("error in (no error)"=w399, "VISA Refnum in"=w404) -> ("error out"=w401:errorcluster, "SR"=w397:string)  [unwired: 7 in, 1 out]
            n145 = Format Into String(Inst.Krohn-Hite-7008.ProtectedCommands--Enum."Set SR" ("Commands")) -> (resulting string=w396:string)  [unwired: 3 in, 1 out]
            n146 = call "Inst.Krohn-Hite-7008.MessageFromProcess.vi"("error in (no error)"=w401, "Data"=w397, "Command"=w396, "Inst.Krohn-Hite-7008 in"=w403) -> ("error out"=w400:errorcluster, "Inst.Krohn-Hite-7008 out"=w402:refnum<class "Inst.Krohn-Hite-7008.lvclass">)  [unwired: 6 in]
            n147 = Bundle By Name(cluster=w405, "SelfRef"=w402) -> (w406:T7)
            n148 = call <vilib>:"Add State(s) to Queue__jki_lib_state_machine.vi"("State(s) in (\"\")"=w409) -> ("States Out"=w408:string)  [unwired: 14 in]
          }
          frame "Instrument: get" {
            n149 = Unbundle By Name(w424) -> ("SelfRef"=w423:refnum<class "Inst.Krohn-Hite-7008.lvclass">, "MessageToProcess.Message.Command"=w416:string, "MessageToProcess.Message.Data"=w417:variant)
            n150 = call "Inst.Krohn-Hite-7008.handleGetCommand.vi"("error in (no error)"=w419, "Data"=w417, "Command in"=w416, "Inst.Krohn-Hite-7008 in"=w423) -> ("error out"=w418:errorcluster, "Data out"=w411:variant, "Command out"=w412:string, "Inst.Krohn-Hite-7008 out"=w422:refnum<class "Inst.Krohn-Hite-7008.lvclass">)  [unwired: 4 in]
            n151 = Empty String/Path?(string/path=w412) -> (empty?=w415:bool)
            n152 = Empty String/Path?(string/path=w411) -> (empty?=w414:bool)
            n153 = Or(x=w415, y=w414) -> (x .or. y?=w413:bool)
            n154 = case shown="False" w413 {
              tunnel: w422 -> [w440 w442]
              tunnel: [w437 w442] -> w421
              tunnel: [w429 w443] -> w420
              tunnel: w418 -> [w439 w443]
              tunnel: w412 -> [_ _]
              tunnel: w411 -> [w438 _]
              tunnel: w411 -> [w434 _]
              tunnel: [w433 ""] -> w410
              frame False {
                n155 = call <userlib>:"setAllData.vi"("error in (no error)"=w439, "AllData"=w438, "Instrument in"=w440) -> ("error out"=w430:errorcluster, "Instrument out"=w437:refnum<class "Inst.Krohn-Hite-7008.lvclass">)  [unwired: 7 in]
                n156 = Variant To Data(error in=w430, Variant=w434) -> (data=w435:T11, error out=w436:errorcluster)  [unwired: 1 in]
                n157 = call "Convert_allChannelProperties_to_JSON.vi"("error in (no error)"=w436, "allChannelProperties"=w435) -> ("error out"=w429:errorcluster, "<JSON>"=w432:string)  [unwired: 8 in]
                n158 = Format Into String(format string="Sequence: Status >> \"%s\"", w432) -> (resulting string=w433:string)  [unwired: 2 in, 1 out]
              }
              frame True {
                # "do not send empty data"
              }
            }
            n159 = Bundle By Name(cluster=w424, "SelfRef"=w421) -> (w425:T7)
            n160 = call <vilib>:"Add State(s) to Queue__jki_lib_state_machine.vi"("State(s) in Front (\"\")"=w410, "State(s) in (\"\")"=w428) -> ("States Out"=w427:string)  [unwired: 13 in]
          }
          frame "Instrument: set" {
            # "confirm settings were saved\n(and also alert UI and other listeners)"
            n161 = Unbundle By Name(w451) -> ("SelfRef"=w450:refnum<class "Inst.Krohn-Hite-7008.lvclass">, "MessageToProcess.Message.Command"=w446:string, "MessageToProcess.Message.Data"=w445:variant)
            n162 = call "Inst.Krohn-Hite-7008.handleSetCommand.vi"("error in (no error)"=w448, "Data"=w445, "Command"=w446, "Inst.Krohn-Hite-7008 in"=w450) -> ("error out"=w447:errorcluster, "Inst.Krohn-Hite-7008 out"=w449:refnum<class "Inst.Krohn-Hite-7008.lvclass">)  [unwired: 6 in]
            n163 = Bundle By Name(cluster=w451, "SelfRef"=w449) -> (w452:T7)
            n164 = call <vilib>:"Add State(s) to Queue__jki_lib_state_machine.vi"("State(s) in Front (\"\")"="Instrument: get" ("State(s) in Front (\"\")"), "State(s) in (\"\")"=w455) -> ("States Out"=w454:string)  [unwired: 13 in]
          }
          frame "Instrument: Log" {
            n165 = Unbundle By Name(w464) -> ("SelfRef"=w458:refnum<class "Inst.Krohn-Hite-7008.lvclass">)
            n166 = Unbundle By Name(w458) -> ("getAll"=w460:T19)
            n167 = Unbundle By Name(w460) -> ("device_id"=w457:string, "allChannelProperties"=w461:T11)
            n168 = for {
              tunnel: w461 -> [w476] mode=indexing
              tunnel: [w469] -> w459
              tunnel: w456 -> [w481]
              tunnel: w458 -> [w480]
              tunnel: [w482] -> w462
              tunnel: w457 -> [w474]
              tunnel: w456 -> [w472]
              n169 = call-dynamic "Get SMO Database Paths.vi"("error in (no error)"=w481, "Inst.Krohn-Hite-7008 in"=w480) -> ("error out"=w479:errorcluster, "Paths"=w478:string, "Inst.Krohn-Hite-7008 out"=w477:refnum<class "Inst.Krohn-Hite-7008.lvclass">)  [unwired: 7 in]
              n170 = call "Convert_ChannelProperty_to_JSON.vi"("error in (no error)"=w472, "channelProperties"=w476) -> ("error out"=w471:errorcluster, "getChannelResponse"=w475:T20)  [unwired: 8 in]
              n171 = Bundle By Name(cluster=w475, "device_id"=w474) -> (w473:T20)
              n172 = call <userlib>:"Instrument.logToDatabase.vi"("error in (no error)"=w479, "Data"=w473, "Paths"=w478, "Instrument"=w477) -> ("error out"=w470:errorcluster, "Instrument out"=w482:refnum<class "Inst.Krohn-Hite-7008.lvclass">)  [unwired: 6 in]
              n173 = Merge Errors(w470, w471) -> (w469:errorcluster)
            }
            n174 = Bundle By Name(cluster=w464, "SelfRef"=w462) -> (w465:T7)
            n175 = call <vilib>:"Add State(s) to Queue__jki_lib_state_machine.vi"("State(s) in Front (\"\")"="" ("State(s) in Front (\"\")"), "State(s) in (\"\")"=w468) -> ("States Out"=w467:string)  [unwired: 13 in]
          }
          frame "Instrument: Close Hardware" {
            n176 = Unbundle By Name(w487) -> ("SelfRef"=w486:refnum<class "Inst.Krohn-Hite-7008.lvclass">)
            n177 = call-dynamic "Close Hardware.vi"("error in (no error)"=w483, "Inst.Krohn-Hite-7008 in"=w486) -> ("error out"=w484:errorcluster, "Inst.Krohn-Hite-7008 out"=w485:refnum<class "Inst.Krohn-Hite-7008.lvclass">)  [unwired: 8 in]
            n178 = Bundle By Name(cluster=w487, "SelfRef"=w485) -> (w488:T7)
            n179 = call <vilib>:"Add State(s) to Queue__jki_lib_state_machine.vi"("State(s) in (\"\")"=w491) -> ("States Out"=w490:string)  [unwired: 14 in]
          }
          frame "---------- Sequence ----------" {
            n180 = call <vilib>:"Add State(s) to Queue__jki_lib_state_machine.vi"("State(s) in (\"\")"=w496) -> ("States Out"=w495:string)  [unwired: 14 in]
          }
          frame "Sequence: Status" {
            # "Sequence: Status\n(Use this frame to pass the status to the UI, this VI's UI, etc)"
            n181 = call <vilib>:"Add State(s) to Queue__jki_lib_state_machine.vi"("State(s) in (\"\")"=w502) -> ("States Out"=w501:string)  [unwired: 14 in]
            "Status" <- w497
          }
          frame "Sequence: Wait" {
            # "Sequence: Wait\n(Non-Blocking Wait)"
            # "F = repeat this state. wait\nT = go to next state. don't wait"
            n182 = Unbundle By Name(w511) -> ("Running Step"=w504:i32)
            n183 = call <userlib>:"Wait Logic.vi"("error in (no error)"=w507, "Time"=w505) -> ("error out"=w506:errorcluster, "Status String"=w503:string, "Trigger"=w508:bool)  [unwired: 6 in, 1 out]
            n184 = Increment(x=w504) -> (x+1=w518:i32)
            n185 = Select(t=w518, s=w508, f=w504) -> (s? t:f=w509:i32)
            n186 = Select(t=u32 0, s=w508, f=u32 100 ("milliseconds to wait")) -> (s? t:f=w515:u32)
            n187 = call <userlib>:"Wait (ms)__ogtk.vi"("error in (no error)"=w506, "milliseconds to wait"=w515) -> ("error out"=w513:errorcluster)  [unwired: 8 in, 1 out]
            n188 = Bundle By Name(cluster=w511, "Running Step"=w509) -> (w510:T7)
            n189 = call <vilib>:"Build State String with Arguments__JKI_lib_State_Machine.vi"("Arguments (\"\")"=w503, "State"="Sequence: Status") -> ("State with Arguments"=w512:string)  [unwired: 4 in]
            n190 = call <vilib>:"Add State(s) to Queue__jki_lib_state_machine.vi"("State(s) in Front (\"\")"=w512, "State(s) in (\"\")"=w521) -> ("States Out"=w520:string)  [unwired: 13 in]
          }
        }
      }
    }
    frame Error {
    }
  }
  n191 = call-parent "Process.vi"("error in"=w5, "Instrument"=w4) -> ("error out"=w2:errorcluster, "Instrument out"=→"Inst.Krohn-Hite-7008 out":refnum<class "Inst.Krohn-Hite-7008.lvclass">)  [unwired: 8 in]
  n192 = Merge Errors(w2, w1) -> (→"error out":errorcluster)
